vi "GEOM_DeleteOverrwcs.vi"(8 "error in (no error)":errorcluster, 9 "curr arr":string[][](array[string]), 10 "extension data":string) -> (0 "error out":errorcluster, 2 "out":string[][](array[string]))   [LabVIEW 2016]
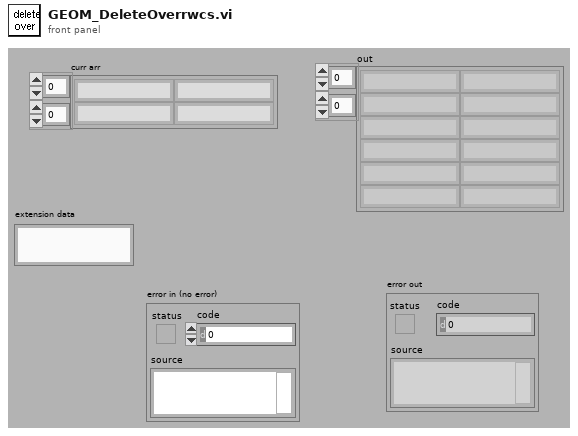
[diagram p1: front panel]
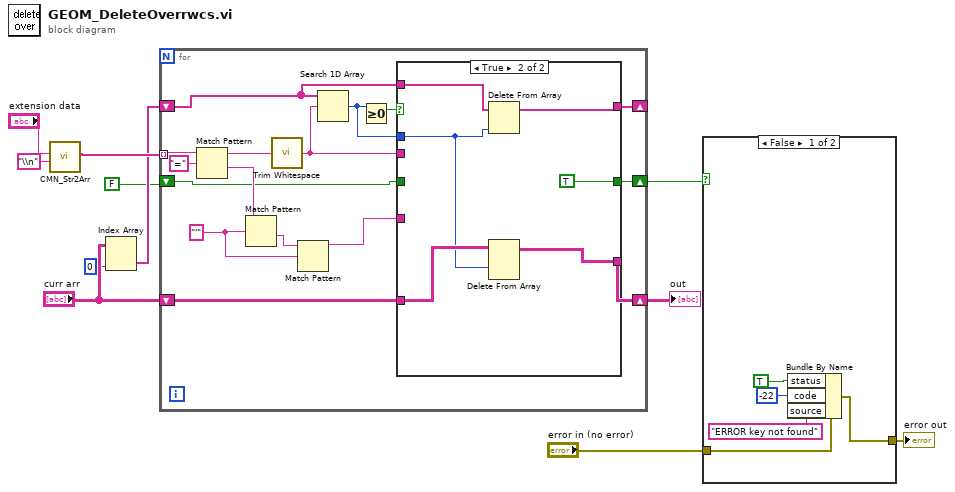
[diagram p0: block diagram]
diagram:
  n1 = call "CMN_Str2Arr.vi"("separator"="\\n", "string in"="extension data") -> ("Array out"=w9:string[])  [unwired: 2 in, 7 out]
  n2 = Index Array(array="curr arr", index (col)=0 ("disabled index (col)")) -> (element=w6:string[])  [unwired: 1 in]
  n3 = for {
    tunnel: w9 -> [w27] mode=indexing
    shift-right: [w18] -> w11
    shift-left: "curr arr" -> [w19]
    shift-right: [w15] -> _
    shift-left: w6 -> [w17]
    shift-right: [w12] -> w2
    shift-left: FALSE -> [w13]
    w23 = "'" ("regular expression")
    n4 = Match Pattern(string=w27, regular expression="=") -> (before substring=w25:string, after substring=w24:string)  [unwired: 3 out]
    n5 = Match Pattern(string=w24, regular expression=w23) -> (after substring=w21:string)  [unwired: 4 out]
    n6 = call <vilib>:"Trim Whitespace.vi"("string"=w25) -> ("trimmed string"=w16:string)  [unwired: 1 in]
    n7 = Match Pattern(string=w21, regular expression=w23) -> (before substring=w22:string)  [unwired: 4 out]
    n8 = Search 1D Array(1D array=w17, element=w16) -> (index of element=w14:i32)  [unwired: 1 out]
    n9 = Greater Or Equal To 0?(x=w14) -> (x >= 0?=w20:bool)
    n10 = case shown="True" w20 {
      tunnel: w22 -> [_ _]
      tunnel: w16 -> [_ _]
      tunnel: w19 -> [w29 w36]
      tunnel: [w29 w35] -> w18
      tunnel: w17 -> [w30 w34]
      tunnel: [w30 w32] -> w15
      tunnel: w14 -> [_ w33]
      tunnel: w13 -> [w28 _]
      tunnel: [w28 TRUE] -> w12
      frame False {
      }
      frame True {
        n11 = Delete From Array(array=w34, index=w33) -> (array with subset deleted=w32:string[])  [unwired: 1 in, 1 out]
        n12 = Delete From Array(array=w36, index (row)=w33) -> (array with subset deleted=w35:string[][])  [unwired: 2 in, 1 out]
      }
    }
  }
  "out" <- w11
  n13 = case shown="False" w2 {
    tunnel: "error in (no error)" -> [w41 w42]
    tunnel: [w40 w42] -> w1
    frame False {
      n14 = Bundle By Name(cluster=w41, "status"=TRUE, "code"=-22, "source"="ERROR key not found") -> (w40:errorcluster)
    }
    frame True {
    }
  }
  "error out" <- w1
